vi "Untitled 4.vi"() -> ()   [LabVIEW 2017]
uses:
  <vilib>/Utility/file.llb/Write Delimited Spreadsheet (DBL).vi
panel:
  in  "millisecond timer value":u32
  in  "stop":bool
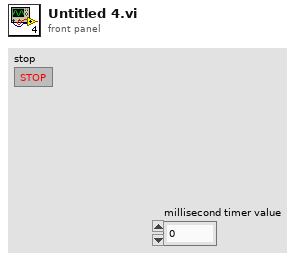
[diagram p1: front panel]
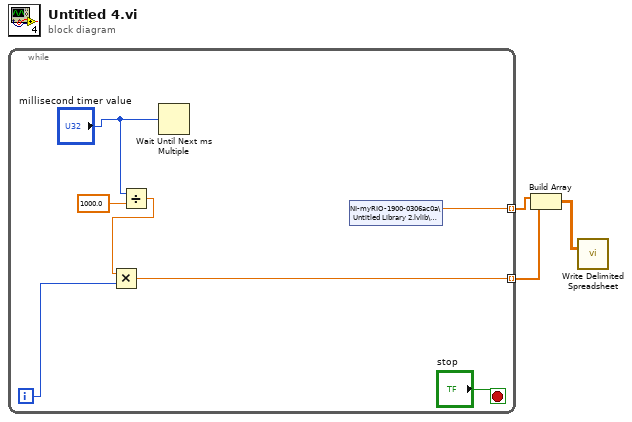
[diagram p0: block diagram]
diagram:
  n1 = while {
    tunnel: [w5] -> w3 mode=indexing
    tunnel: [w4] -> w2 mode=indexing
    i -> [w7]
    stop <- "stop" stop-if-true
    n2 = Divide(x="millisecond timer value", y=1000.0) -> (x/y=w6:dbl)
    n3 = Multiply(x=w6, y=w7) -> (x*y=w4:dbl)
    n4 = Wait Until Next ms Multiple(millisecond multiple="millisecond timer value") -> ()  [unwired: 1 out]
    n5 = shared-variable "NI-myRIO-1900-0306ac0a\\Untitled Library 2.lvlib\\Variable1"() -> (w5:dbl)  [unwired: 1 in, 1 out]
  }
  n6 = Build Array(w3, w2) -> (w1:dbl[][])
  n7 = call-poly <vilib>:"Write Delimited Spreadsheet.vi"("2D data"=w1) -> ()  [unwired: 13 in, 2 out]
